vi "set_settings_to_controls.vi"(8 "error in (no error)":errorcluster, 11 "TrajectoryMH100122AODRAPS in":refnum<class "TrajectoryMH100122AODRAPS.lvclass">) -> (0 "error out":errorcluster, 3 "TrajectoryMH100122AODRAPS out":refnum<class "TrajectoryMH100122AODRAPS.lvclass">)   [LabVIEW 2010, in "TrajectoryMH100122AODRAPS.lvclass"]
uses:
  TrajectoryMH100122AODRAPS.lvclass
  TrajectoryMH100122AODRAPS.lvclass/TrajectoryMH100122AODRAPS.ctl
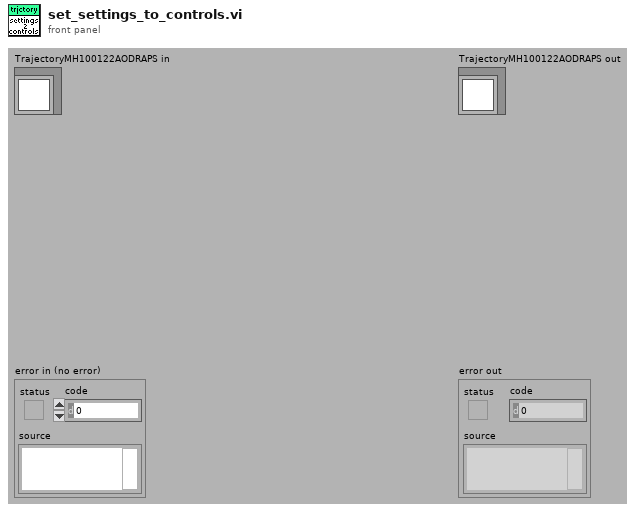
[diagram p1: front panel]
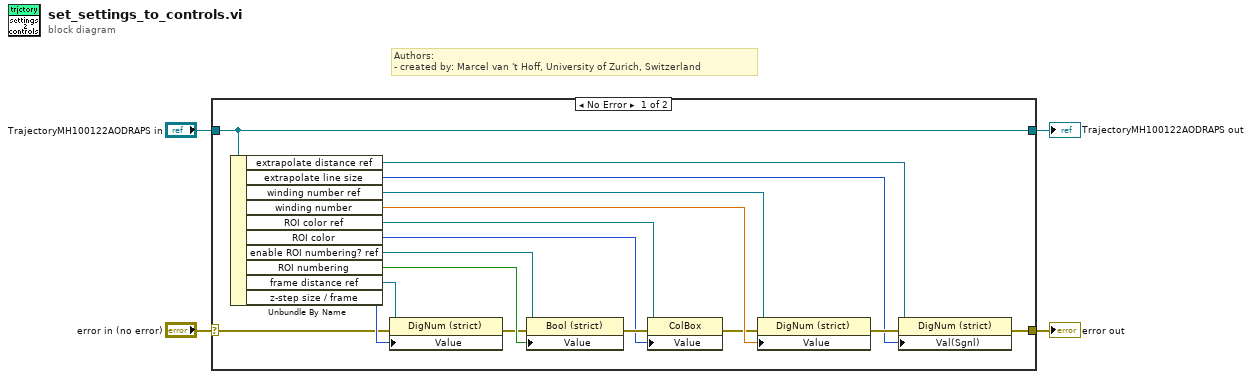
[diagram p0: block diagram]
diagram:
  # "Authors: \n- created by: Marcel van 't Hoff, University of Zurich, Switzerland"
  n1 = case shown="No Error" "error in (no error)" {
    selector: "error in (no error)" -> [w12 w23]
    tunnel: [w8 w23] -> w3
    tunnel: [w21 w22] -> w1
    tunnel: "TrajectoryMH100122AODRAPS in" -> [w21 w22]
    frame No Error {
      n2 = Unbundle By Name(w21) -> ("extrapolate distance ref"=w10:refnum<vi>, "extrapolate line size"=w6:i32, "winding number ref"=w11:refnum<vi>, "winding number"=w7:dbl, "ROI color ref"=w14:refnum<vi>, "ROI color"=w13:u32, "enable ROI numbering? ref"=w18:refnum<vi>, "ROI numbering"=w17:bool, "frame distance ref"=w20:refnum<vi>, "z-step size / frame"=w19:u16)
      n3 = property class="DigNum (strict)"(reference=w20, error in=w12, "Value"=w19) -> (error out=w16:errorcluster)  [unwired: 1 out]
      n4 = property class="Bool (strict)"(reference=w18, error in=w16, "Value"=w17) -> (error out=w15:errorcluster)  [unwired: 1 out]
      n5 = property class="ColBox"(reference=w14, error in=w15, "Value"=w13) -> (error out=w5:errorcluster)  [unwired: 1 out]
      n6 = property class="DigNum (strict)"(reference=w11, error in=w5, "Value"=w7) -> (error out=w9:errorcluster)  [unwired: 1 out]
      n7 = property class="DigNum (strict)"(reference=w10, error in=w9, "Val(Sgnl)"=w6) -> (error out=w8:errorcluster)  [unwired: 1 out]
    }
    frame Error {
    }
  }
  "error out" <- w3
  "TrajectoryMH100122AODRAPS out" <- w1
